vi "GEN_Histo_Bins_And_X_axis.vi"(8 "Error In":errorcluster, 11 "Histogram parameters":T1={"max"=300.0, "min"=0.0, "# bins"=10, "threshold"=8.0, "thr. type"=enum."higher accepted"}) -> (0 "Error Out":errorcluster, 1 "Initial bins count":u32[](array[numeric]), 2 "Bins":dbl[](array[numeric]), 3 "X axis values":dbl[](array[numeric]))   [LabVIEW 2018, in "Tracker.lvlib"]
uses:
  Tracker.lvlib
  Controls/CTL_Histogram_parameters.ctl
  Common_Resources.lvlib
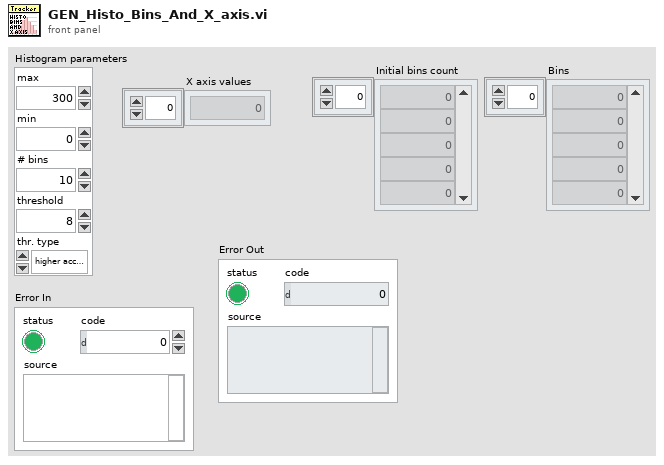
[diagram p1: front panel]
types:
  T1 = typedef "Common_Resources.lvlib/CTL_Histogram_parameters.ctl" = cluster{"max":dbl, "min":dbl, "# bins":i32, "threshold":dbl, "thr. type":enum16{"higher accepted", "lower accepted"}}
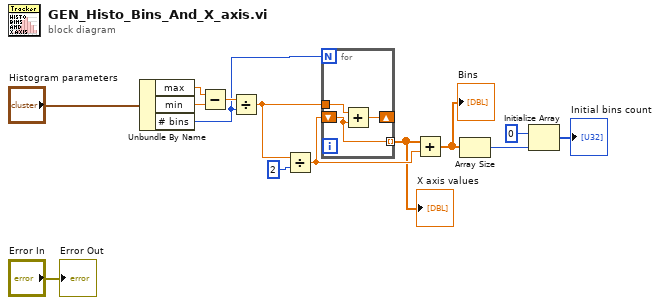
[diagram p0: block diagram]
diagram:
  n1 = Unbundle By Name("Histogram parameters") -> ("max"=w3:dbl, "min"=w2:dbl, "# bins"=w1:i32)
  n2 = Subtract(x=w3, y=w2) -> (x-y=w10:dbl)
  n3 = Divide(x=w10, y=w1) -> (x/y=w12:dbl)
  n4 = Divide(x=w12, y=2) -> (x/y=w14:dbl)
  n5 = for {
    N: w1 -> [_]
    tunnel: w12 -> [w17]
    tunnel: [w15] -> w13 mode=indexing
    shift-right: [w16] -> _
    shift-left: w14 -> [w15]
    n6 = Add(x=w17, y=w15) -> (x+y=w16:dbl)
  }
  "X axis values" <- w13
  n7 = Add(x=w13, y=w14) -> (x+y=w7:dbl[])
  "Bins" <- w7
  n8 = Array Size(array=w7) -> (size(s)=w8:i32)
  n9 = Initialize Array(0, w8) -> (→"Initial bins count":i32[])
  "Error Out" <- "Error In"
